vi "OpenSubpanel.vi"(8 "error in (no error)":errorcluster, 10 "Panel Index":i32, 11 "SMO.UI.MAUI in":refnum<class "SMO.UI.MAUI.lvclass">) -> (0 "error out":errorcluster, 3 "SMO.UI.MAUI out":refnum<class "SMO.UI.MAUI.lvclass">)   [LabVIEW 2019, in "SMO.UI.MAUI.lvclass"]
uses:
  SMO.UI.MAUI.lvclass
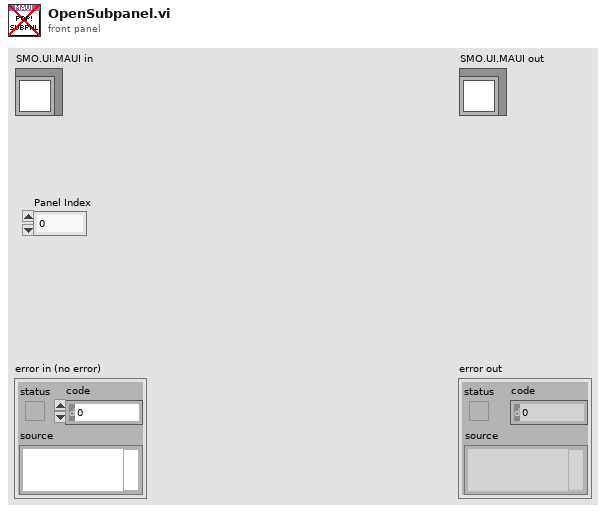
[diagram p1: front panel]
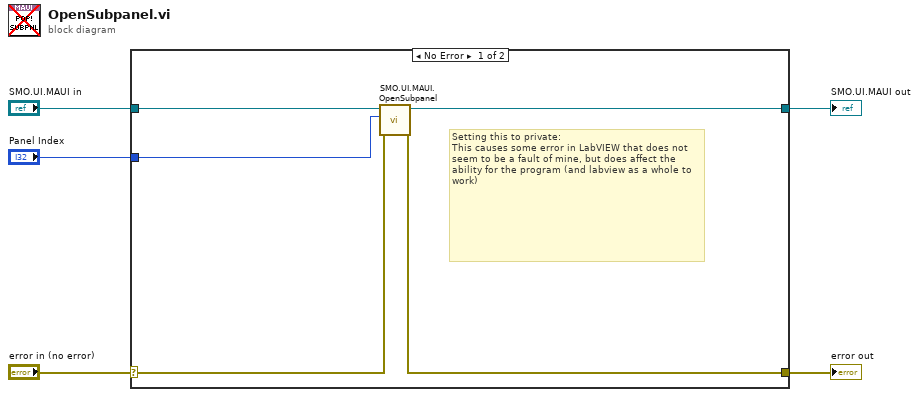
[diagram p0: block diagram]
diagram:
  n1 = case shown="No Error" "error in (no error)" {
    selector: "error in (no error)" -> [w10 w12]
    tunnel: [w9 w12] -> w4
    tunnel: [w7 w11] -> w2
    tunnel: "SMO.UI.MAUI in" -> [w6 w11]
    tunnel: "Panel Index" -> [w8 _]
    frame No Error {
      # "Setting this to private:\nThis causes some error in LabVIEW that does not seem to be a fault of mine, but does affect the ability for the program (and labview as a whole to work)"
      n2 = call "SMO.UI.MAUI.OpenSubpanel.vi"("error in (no error)"=w10, "OpenSubpanel"=w8, "SMO.UI.MAUI"=w6) -> ("error out"=w9:errorcluster, "SMO.UI.MAUI out"=w7:refnum<class "SMO.UI.MAUI.lvclass">)  [unwired: 7 in]
    }
    frame Error {
    }
  }
  "error out" <- w4
  "SMO.UI.MAUI out" <- w2
